vi "Keith 7001 Perform Scan.vi"(0 "GPIB address":string="7", 1 "error in":T1, 2 "scan options (arm, scan once:0)":u16(ring) items=["arm, scan channels in scan list once", "arm, scan channels in scan list continuously", "abort scan, go to idle state"], 3 "scan list":T2(array[cluster]) {"column" min=1; "channel/row" min=1; "slot/memory" min=1}) -> (4 "error out":T1)   [LabVIEW 2019]
doc: "This VI for the Keithley 7001 Switch System is used to enter a scan list and start or stop a scan.\n Example scan lists are as follows:\n\n 1!1,2!5 Slot 1, Channel 1 & Slot 2, Channel 2\n 2!2:2!13 Slot 2, Channels 2-13\n 1!14,M12 Slot 1, Channel 14 & Channels at M12"
panel:
  # "memory location\nstandard channel"
  # "matrix card\nnon-matrix card"
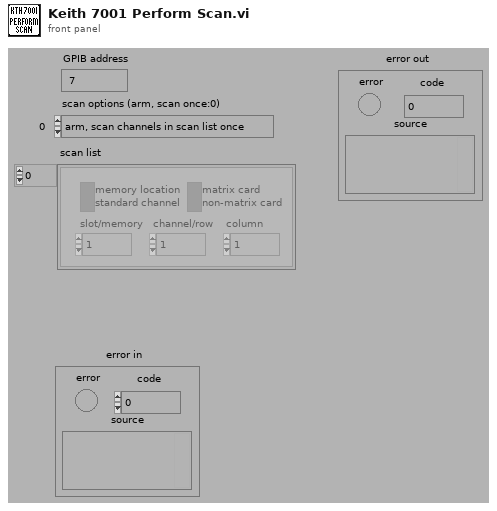
[diagram p1: front panel]
types:
  T1 = cluster{"error":bool, "code":i32, "source":string}
  T2 = cluster{"slot/memory":i16, "channel/row":i16, "column":i16, bool, bool}[]
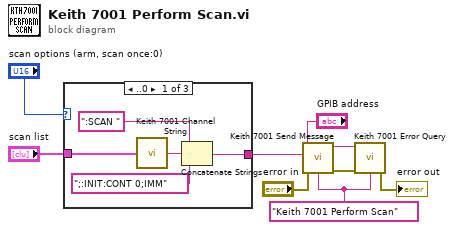
[diagram p0: block diagram]
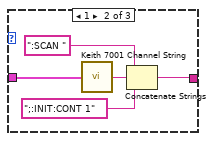
[diagram p2: hidden frame]
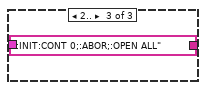
[diagram p3: hidden frame]
diagram:
  w2 = "Keith 7001 Perform Scan"
  n1 = case shown="..0" "scan options (arm, scan once:0)" {
    tunnel: "scan list" -> [w11 w15 _]
    tunnel: [w12 w17 ":INIT:CONT 0;:ABOR;:OPEN ALL"] -> w7
    frame ..0 {
      n2 = call "Keith 7001 Channel String.vi"("channel list"=w11) -> (0:w10:string)
      n3 = Concatenate Strings(":SCAN ", w10, ";:INIT:CONT 0;IMM") -> (w12:string)
    }
    frame 1 {
      n4 = call "Keith 7001 Channel String.vi"("channel list"=w15) -> (0:w16:string)
      n5 = Concatenate Strings(":SCAN ", w16, ";:INIT:CONT 1") -> (w17:string)
    }
    frame 2.. {
    }
  }
  n6 = call "Keith 7001 Send Message.vi"("address string"="GPIB address", "write buffer"=w7, "source"=w2, "error in"="error in") -> ("address out"=w4:string, "error out"=w3:T1)  [unwired: 2 in, 2 out]
  n7 = call "Keith 7001 Error Query.vi"("GPIB address"=w4, "error in"=w3, "source"=w2) -> ("error out"=→"error out":T1)  [unwired: 2 out]
